vi "Stream.Initialize.vi"(8 "error in (no error)":errorcluster, 11 "Parameters":T6={"Name"="", "CAN"={"Interface"="", "Baud Rate"=0, "Diagnostic Protocol"=enum."GMLAN", "Transport Protocol"=enum."ISO TP - Normal Mode", "Transmit ID"=0, "Receive ID"=2, "Transmit Extension"=1, "Receive Extension"=255, "Receive UUDT ID"=0, "Enable Stream"=TRUE, "VW TP Channel ID"=1, "Fill Frame"=FALSE, "Fill Byte"=0, "Termination"=FALSE, "LIN Cluster"="", "NAD"=8, "IO Mode"=0, "Max DLC"=0, "FD Baud Rate"=2, "Timeout"=1, "FD ISO Mode"=0, "DoIP Address"="", "DoIP Source Address"=3584, "DoIP Dynamic Port"=TRUE, "DoIP Version"=2}, "986x"={"Enable"=FALSE, "RIO Device"="", "Bitfile"=path ""}, "Reads"=[], "Frames Lookup"=variant(enum16{"GMLAN", "KWP-2000", "UDS"} enum."GMLAN"), "Writes"=[], "DPIDs"=[], "DPID Lookup"=variant(u32 0), "DTC"={"Descriptor"={"DTC Byte Length"=1, "Status Byte Length"=1, "Add Data Byte Length"=1, "Byte Order"=enum."Motorola"}, "Value.Code"=[], "Value.String"=[], "Value.J2012String"=[], "Status.Code"=[], "Status.String"=[]}, "Created DTCs"=0, "Polls"=[], "Service Channels Status Lookup"=variant, "Trigger Lookup"=variant, "Security"={"Type"=enum."None", "Source DLL Path"=path "", "Target DLL Path"=path "", "Security Level"=0, "Static Master Key"="", "Max Key Length"=1, "Host IP Address"="", "ECU  Variant"=0, "Optional Parameter"=0}, "Initial Comm State"=FALSE} {"Writes"."Signals"."Byte Order" items=["Little Endian", "Big Endian"]; "Writes"."Signals"."Data Type" items=["Signed", "Unsigned", "IEEE Float"]; "CAN"."DoIP Version" items=["2010"=1, "2012"=2]; "CAN"."DoIP Source Address" format="%.0x"; "CAN"."FD ISO Mode" items=["ISO", "Non ISO", "ISO Legacy"]; "CAN"."IO Mode" items=["CAN 2.0", "CAN FD", "CAN FD+BRS"]; "CAN"."Fill Byte" format="%.0x"; "CAN"."VW TP Channel ID" format="%.0x"; "CAN"."Receive UUDT ID" format="%.0x"; "CAN"."Receive Extension" format="%.0x"; "CAN"."Transmit Extension" format="%.0x"; "CAN"."Receive ID" format="%.0x"; "CAN"."Transmit ID" format="%.0x"; "Reads"."Signals"."Byte Order" items=["Little Endian", "Big Endian"]; "Reads"."Signals"."Data Type" items=["Signed", "Unsigned", "IEEE Float"]}) -> (0 "error out":errorcluster, 3 "Stream Refs":T1 {"Port Settings"."FD ISO Mode" items=["ISO", "Non ISO", "ISO Legacy"]; "Port Settings"."Termination" items=["Off", "On"]; "Port Settings"."Mode" items=["CAN 2.0", "CAN FD", "CAN FD+BRS"]})   [LabVIEW 2024, in "Diagnostics Addon Engine.lvlib"]
uses:
  Diagnostics Addon Engine.lvlib
  Addon Shared/Types/SysDef.Compile.ctl
  Addon Shared/Types/CAN.ctl
  Addon Shared/Types/CAN.Interface.ctl
  Addon Shared/Types/Protocol.ctl
  Addon Shared/Types/Transport.ctl
  Addon Shared/Types/986x.ctl
  Addon Shared/Types/Frame.Compile.ctl
  Addon Shared/Types/Type.ctl
  Addon Shared/Types/Signal.ctl
  Addon Shared/Types/DPID.ctl
  Addon Shared/Types/DPID.Rate.ctl
  Addon Shared/Types/DTC.Settings.ctl
  Addon Shared/Types/DTC.Descriptor.ctl
  Addon Shared/Types/Poll.Compiled.ctl
  Addon Shared/Types/Security.ctl
  Addon Shared/Types/Security.Type.ctl
  SubModules/CAN-Streaming-Support/Source/Addon/Addon Engine/Types/Engine Stream Refs.ctl
  SubModules/CAN-Streaming-Support/Source/Addon/Addon Shared/Types/Direction Filter.ctl
  SubModules/CAN-Streaming-Support/Source/Addon/Addon Shared/Types/Type Filter.ctl
  SubModules/CAN-Streaming-Support/Source/Addon/Addon Shared/Types/Filter Parameters.ctl
  SubModules/CAN-Streaming-Support/Source/Addon/Addon Engine/Types/Engine Stream Port Settings.ctl
  SubModules/CAN-Streaming-Support/Source/Addon/Addon Engine/CAN Stream Support Engine.lvlib
  Addon Shared/Diagnostics Addon Shared.lvlib
  SubModules/CAN-Streaming-Support/Source/Addon/Addon Shared/CAN Stream Support Shared.lvlib
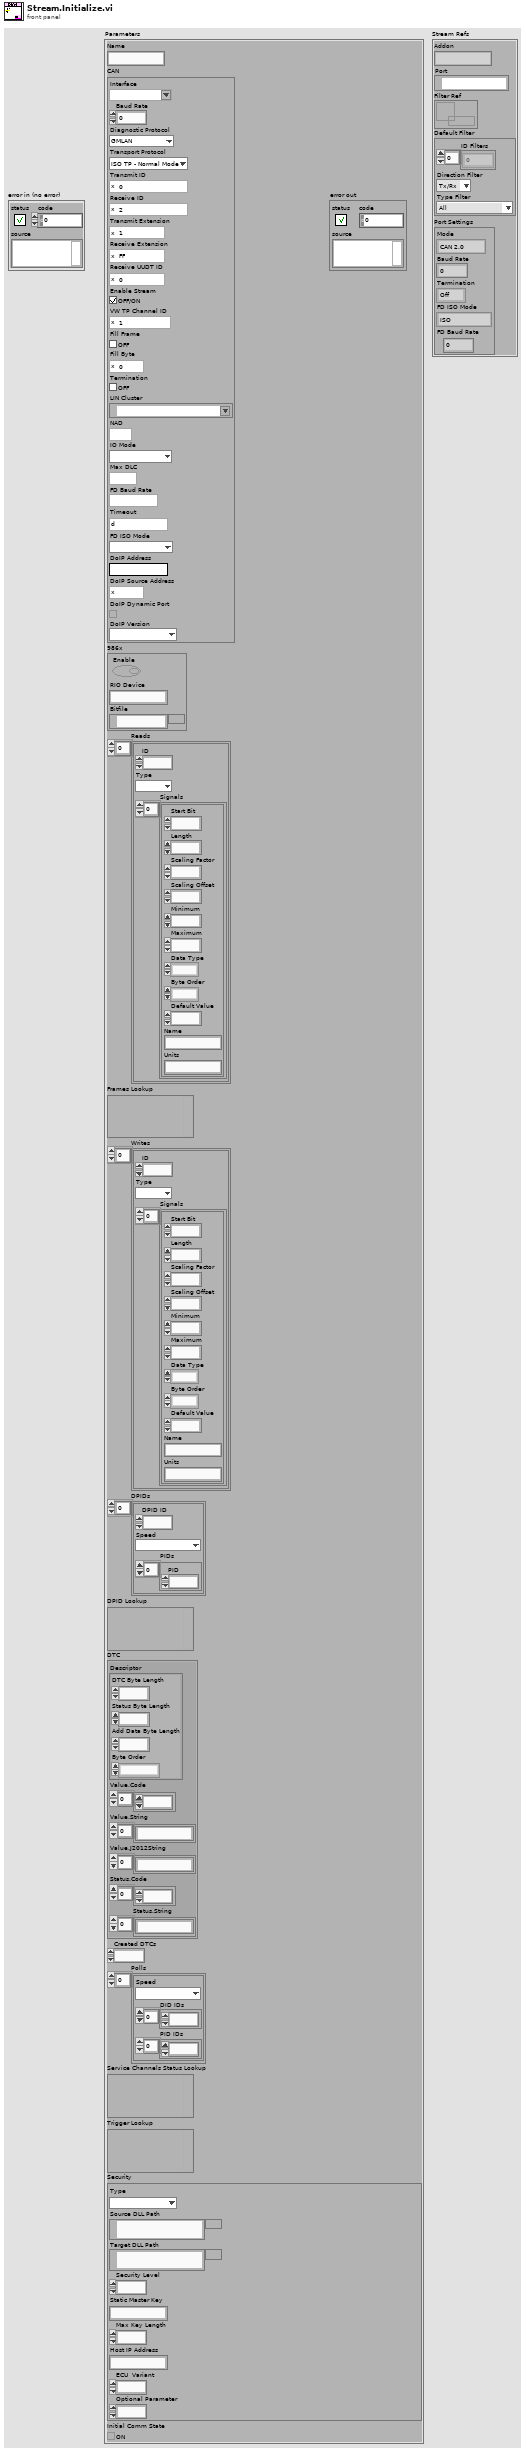
[diagram p1: front panel]
types:
  T1 = typedef "CAN Stream Support Engine.lvlib/Engine Stream Refs.ctl" = cluster{"Addon":string, "Port":refnum<k21>, "Filter Ref":refnum<data-value>, "Default Filter":T2, "Port Settings":T5}
  T2 = typedef "CAN Stream Support Shared.lvlib/Filter Parameters.ctl" = cluster{"ID Filters":u32[], "Direction Filter":T3, "Type Filter":T4}
  T3 = typedef "CAN Stream Support Shared.lvlib/Direction Filter.ctl" = enum16{"Tx/Rx", "Rx", "Tx"}
  T4 = typedef "CAN Stream Support Shared.lvlib/Type Filter.ctl" = enum16{"All", "CAN Data", "CAN Remote", "CAN Bus Error", "CAN 2.0 Data", "CAN FD Data", "CAN FD+BRS Data", "J1939 Data", "Delay", "Log Trigger", "Start Trigger"}
  T5 = typedef "CAN Stream Support Engine.lvlib/Engine Stream Port Settings.ctl" = cluster{"Mode":u32, "Baud Rate":u64, "Termination":u32, "FD ISO Mode":u32, "FD Baud Rate":u64}
  T6 = typedef "Diagnostics Addon Shared.lvlib/SysDef.Compile.ctl" = cluster{"Name":string, "CAN":T7, "986x":T11, "Reads":T12[], "Frames Lookup":variant, "Writes":T12[], "DPIDs":T15[], "DPID Lookup":variant, "DTC":T17, "Created DTCs":u32, "Polls":T19[], "Service Channels Status Lookup":variant, "Trigger Lookup":variant, "Security":T20, "Initial Comm State":bool}
  T7 = typedef "Diagnostics Addon Shared.lvlib/CAN.ctl" = cluster{"Interface":T8, "Baud Rate":u64, "Diagnostic Protocol":T9, "Transport Protocol":T10, "Transmit ID":u32, "Receive ID":u32, "Transmit Extension":u8, "Receive Extension":u8, "Receive UUDT ID":u32, "Enable Stream":bool, "VW TP Channel ID":u32, "Fill Frame":bool, "Fill Byte":u8, "Termination":bool, "LIN Cluster":refnum<k21>, "NAD":u8, "IO Mode":u32, "Max DLC":u16, "FD Baud Rate":u64, "Timeout":u32, "FD ISO Mode":u32, "DoIP Address":string, "DoIP Source Address":u16, "DoIP Dynamic Port":bool, "DoIP Version":u16}
  T8 = typedef "Diagnostics Addon Shared.lvlib/CAN.Interface.ctl" = string
  T9 = typedef "Diagnostics Addon Shared.lvlib/Protocol.ctl" = enum16{"GMLAN", "KWP-2000", "UDS", "User-Defined"}
  T10 = typedef "Diagnostics Addon Shared.lvlib/Transport.ctl" = enum16{"ISO TP - Normal Mode", "ISO TP - Mixed Mode", "VW TP 2.0", "Diagnostics on IP", "ISO TP LIN"}
  T11 = typedef "Diagnostics Addon Shared.lvlib/986x.ctl" = cluster{"Enable":bool, "RIO Device":string, "Bitfile":path}
  T12 = typedef "Diagnostics Addon Shared.lvlib/Frame.Compile.ctl" = cluster{"ID":u32, "Type":T13, "Signals":T14[]}
  T13 = typedef "Diagnostics Addon Shared.lvlib/Type.ctl" = enum16{"DID", "CDID", "PID", "CPID", "Read Memory", "Write Memory", "IO Control", "Routine Start", "Routine Request", "Routine Stop", "User Defined", "DTC Control", "Clear DTCs", "Read DTCs", "Start DTCs", "DTC Change Count", "Tester Present", "Unlock ECU", "Reset ECU", "Diag Session Control", "Communication Control", "DPID Control", "Poll Control", "Diag Comm Port Control"}
  T14 = typedef "Diagnostics Addon Shared.lvlib/Signal.ctl" = cluster{"Start Bit":u32, "Length":u32, "Scaling Factor":dbl, "Scaling Offset":dbl, "Minimum":dbl, "Maximum":dbl, "Data Type":u32, "Byte Order":u32, "Default Value":dbl, "Name":string, "Units":string}
  T15 = typedef "Diagnostics Addon Shared.lvlib/DPID.ctl" = cluster{"DPID ID":u8, "Speed":T16, "PIDs":u16[]}
  T16 = typedef "Diagnostics Addon Shared.lvlib/DPID.Rate.ctl" = enum16{"Slow", "Medium", "Fast"}
  T17 = typedef "Diagnostics Addon Shared.lvlib/DTC.Settings.ctl" = cluster{"Descriptor":T18, "Value.Code":dbl[], "Value.String":string[], "Value.J2012String":string[], "Status.Code":dbl[], "Status.String":string[]}
  T18 = typedef "Diagnostics Addon Shared.lvlib/DTC.Descriptor.ctl" = cluster{"DTC Byte Length":i32, "Status Byte Length":i32, "Add Data Byte Length":i32, "Byte Order":enum16{"Motorola", "Intel"}}
  T19 = typedef "Diagnostics Addon Shared.lvlib/Poll.Compiled.ctl" = cluster{"Speed":T16, "DID IDs":u32[], "PID IDs":u32[]}
  T20 = typedef "Diagnostics Addon Shared.lvlib/Security.ctl" = cluster{"Type":T21, "Source DLL Path":path, "Target DLL Path":path, "Security Level":u32, "Static Master Key":string, "Max Key Length":u32, "Host IP Address":string, "ECU  Variant":i8, "Optional Parameter":i8}
  T21 = typedef "Diagnostics Addon Shared.lvlib/Security.Type.ctl" = enum16{"None", "SeedKey DLL", "MasterKey (Channel)", "MasterKey (Static)", "SeedKey DLL (Windows)"}
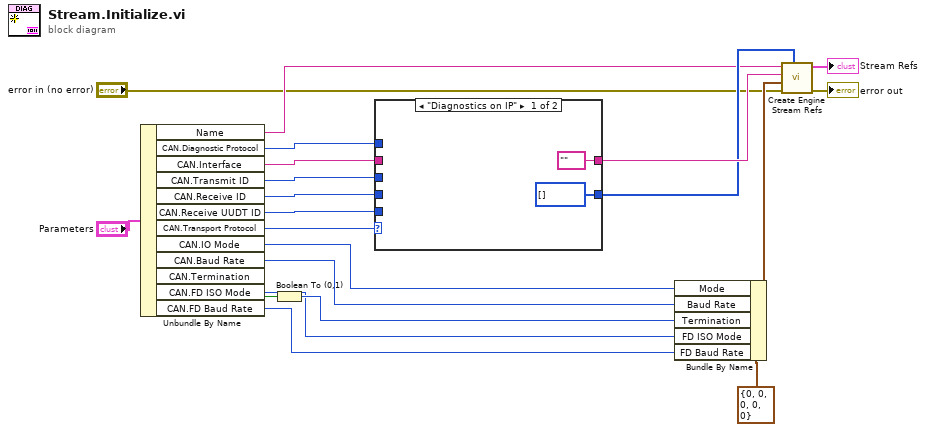
[diagram p0: block diagram]
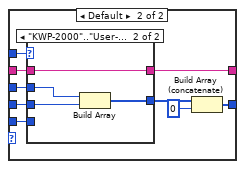
[diagram p2: hidden frame]
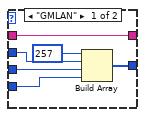
[diagram p3: hidden frame]
diagram:
  n1 = Unbundle By Name("Parameters") -> ("Name"=w3:string, "CAN.Diagnostic Protocol"=w4:T9, "CAN.Interface"=w5:T8, "CAN.Transmit ID"=w19:u32, "CAN.Receive ID"=w18:u32, "CAN.Receive UUDT ID"=w17:u32, "CAN.Transport Protocol"=w1:T10, "CAN.IO Mode"=w10:u32, "CAN.Baud Rate"=w9:u64, "CAN.Termination"=w14:bool, "CAN.FD ISO Mode"=w6:u32, "CAN.FD Baud Rate"=w7:u64)
  n2 = Boolean To (0,1)(Boolean=w14) -> (0, 1=w8:i16)
  n3 = case shown="\"Diagnostics on IP\"" w1 {
    tunnel: [T8 "" ("Interface") w32] -> w20
    tunnel: w19 -> [_ w31]
    tunnel: w18 -> [_ w30]
    tunnel: w17 -> [_ w29]
    tunnel: [u32[] [] w26] -> w13
    tunnel: w5 -> [_ w25]
    tunnel: w4 -> [_ w24]
    frame "Diagnostics on IP" {
    }
    frame Default {
      n4 = case shown="\"KWP-2000\"..\"User-Defined\"" w24 {
        tunnel: w25 -> [w38 w42]
        tunnel: [w38 w42] -> w32
        tunnel: w31 -> [w37 w41]
        tunnel: w30 -> [w36 w40]
        tunnel: w29 -> [w35 _]
        tunnel: [w34 w39] -> w27
        frame "GMLAN" {
          n5 = Build Array(u32 257 ("element"), w37, w36, w35) -> (w34:u32[])
        }
        frame "KWP-2000".."User-Defined" {
          n6 = Build Array(w41, w40) -> (w39:u32[])
        }
      }
      n7 = Build Array (concatenate)(w27, u32 0) -> (w26:u32[])
    }
  }
  n8 = Bundle By Name(cluster=T5 {"Mode"=0, "Baud Rate"=0, "Termination"=0, "FD ISO Mode"=0, "FD Baud Rate"=0} ("Port Settings"), "Mode"=w10, "Baud Rate"=w9, "Termination"=w8, "FD ISO Mode"=w6, "FD Baud Rate"=w7) -> (w11:T5)
  n9 = call "Create Engine Stream Refs.vi"("Default IDs"=w13, "error in (no error)"="error in (no error)", "Port Settings"=w11, "Port"=w20, "Addon"=w3) -> ("error out"=→"error out":errorcluster, "Refs"=→"Stream Refs":T1)  [unwired: 5 in]
